vi "SubVI_Example_Get_AutoFeatures_Sensor_GainShutter.vi"(7 "error in (no error)":errorcluster, 10 ".NET (Reference)":refnum<k24>) -> (0 "error out":errorcluster, 2 "Enabled":bool, 3 "Supported":bool)   [LabVIEW 2016]
uses:
  C:/Program Files/National Instruments/LabVIEW 2016/instr.lib/IDS/ueye.NET/uEyeDotNet.dll
  Program Files/National Instruments/LabVIEW 2016/instr.lib/IDS/ueye.NET/uEyeDotNet.dll
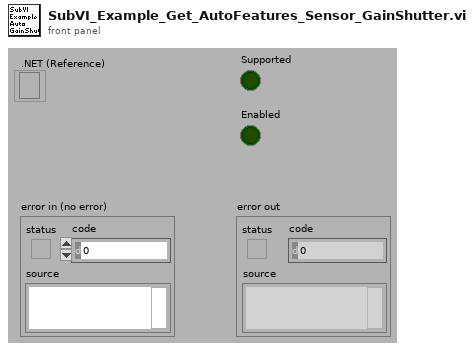
[diagram p1: front panel]
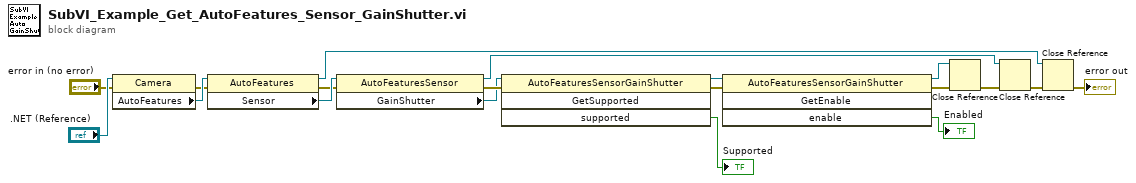
[diagram p0: block diagram]
diagram:
  n1 = property class="Camera"(reference=".NET (Reference)", error in="error in (no error)") -> (error out=w16:errorcluster, "AutoFeatures"=w17:refnum<k24>)  [unwired: 1 out]
  n2 = property class="AutoFeatures"(reference=w17, error in=w16) -> (reference out=w12:refnum<k24>, error out=w14:errorcluster, "Sensor"=w15:refnum<k24>)
  n3 = property class="AutoFeaturesSensor"(reference=w15, error in=w14) -> (reference out=w13:refnum<k24>, error out=w7:errorcluster, "GainShutter"=w1:refnum<k24>)
  n4 = invoke class="AutoFeaturesSensorGainShutter" method="GetSupported"(reference=w1, error in=w7) -> (reference out=w4:refnum<k24>, error out=w6:errorcluster, "supported"=→"Supported":bool)  [unwired: 2 in, 1 out]
  n5 = invoke class="AutoFeaturesSensorGainShutter" method="GetEnable"(reference=w4, error in=w6) -> (reference out=w3:refnum<k24>, error out=w2:errorcluster, "enable"=→"Enabled":bool)  [unwired: 2 in, 1 out]
  n6 = Close Reference(reference=w3, error in (no error)=w2) -> (error out=w9:errorcluster)
  n7 = Close Reference(reference=w13, error in (no error)=w9) -> (error out=w11:errorcluster)
  n8 = Close Reference(reference=w12, error in (no error)=w11) -> (error out=→"error out":errorcluster)
